vi "Back up values.vi"() -> ()   [LabVIEW 2017]
uses:
  Global/GPIB Type Def.ctl
panel:
  in  "Keithley Values":T1={"range (auto:0)"=0, "range value (volts)"=1000.0, "resolution (4.5 digits:3)"=3, "integration time (0:auto)"=0, "integ. value"=0.01667, "digital filter (off:0)"=0, "advanced filter (off:0)"=0, "dig. filter count"=10.0, "reference (off:0)"=0, "reference value (volts)"=0.0, "noise tolerance (%)"=1.0} {"noise tolerance (%)" min=0.0 max=100.0 step=1.0 format="%^.2e"; "reference value (volts)" min=-1100.0 max=1100.0 format="%^.2e"; "reference (off:0)" items=["off", "set reference value"]; "dig. filter count" min=1.0 max=100.0 step=1.0 format="%^.2e"; "advanced filter (off:0)" items=["off", "enabled"]; "digital filter (off:0)" items=["off", "auto filter", "auto filter once", "moving filter", "repeating filter"]; "integ. value" format="%^.2e"; "integration time (0:auto)" items=["automatic", "automatic once", "set to minimum", "set to maximum", "set aperature value", "set NPLC value"]; "resolution (4.5 digits:3)" items=["auto resolution", "auto resolution once", "3.5 digits", "4.5 digits", "5.5 digits", "6.5 digits", "7.5 digits", "8.5 digits"]; "range (auto:0)" items=["autorange", "autorange once", "set min range", "set max range", "set range value"]; "range value (volts)" min=0.2 max=1000.0 format="%^.2e"}
  in  "Cluster of class private data":T3={"Keithley Multimeter"={"Name"="Keithley Multimeter", "bus"=0.0, "GPIB"=18.0, "GPIB as string"="18", "byte"=1024, "VISA Resource Name"="GPIB0::18::INSTR"}, "Configuration Values"={"range (auto:0)"=0, "dig. filter count"=10.0, "digital filter (off:0)"=0, "advanced filter (off:0)"=0, "integration time (0:auto)"=0, "integ. value"=0.01667, "resolution (4.5 digits:3)"=3, "noise tolerance (%)"=1.0, "reference (off:0)"=0, "coupling"=TRUE, "function (Vdc:1)"=1}, "Frequency Configuration"={"source"=FALSE, "resolution (5 digits:1)"=1, "threshold current range (1mA:0)"=0, "reference value (Hz)"=0.0, "threshold current level"=0.0, "threshold voltage range (10V:1)"=1, "threshold voltage level"=0.0}, "DC Current Configuration"={"reference value (amps)"=0.0, "method"=TRUE, "range value (amps)"=2.0}, "AC Current Configuration"={"detector (rms:0)"=0, "reference value (amps)"=0.0, "range value (amps)"=2.0}, "4 Wire Resistance Configuration"={"offset compensation"=FALSE, "reference value (ohms)"=0.0, "range value (ohms)"=200000.0}, "2 Wire Resistance Configuration"={"offset compensation"=FALSE, "reference value (ohms)"=0.0, "range value (ohms)"=1000000000.0}, "DC Voltage Configuration"={"reference value (volts)"=0.0, "range value (volts)"=1000.0}, "AC Voltage Configuration"={"dBm ref impedance (75:1)"=1, "peak window (secs)"=0.1, "detector (rms:0)"=0, "dB reference (volts)"=1.0, "AC voltage (volts:0)"=0, "reference value (volts)"=0.0, "range value (volts)"=750.0}} {"AC Voltage Configuration"."range value (volts)" min=0.2 max=750.0 format="%^.2e"; "AC Voltage Configuration"."reference value (volts)" min=-775.0 max=775.0 format="%^.2e"; "AC Voltage Configuration"."AC voltage (volts:0)" items=["volts", "DB", "DBM"]; "AC Voltage Configuration"."dB reference (volts)" min=0.001 max=750.0 format="%.3f"; "AC Voltage Configuration"."detector (rms:0)" items=["RMS", "average", "low frequency RMS", "AC peak voltage", "DC negative peak spike", "DC positive peak spike"]; "AC Voltage Configuration"."peak window (secs)" min=0.1 max=9.9 format="%.2f"; "AC Voltage Configuration"."dBm ref impedance (75:1)" items=["50 ohms", "75 ohms", "93 ohms", "132 ohms", "300 ohms", "600 ohms"]; "DC Voltage Configuration"."range value (volts)" min=0.2 max=1000.0 format="%^.2e"; "DC Voltage Configuration"."reference value (volts)" min=-1100.0 max=1100.0 format="%^.2e"; "2 Wire Resistance Configuration"."range value (ohms)" min=20.0 max=1000000000.0 format="%^.2e"; "2 Wire Resistance Configuration"."reference value (ohms)" min=-1000000000.0 max=1000000000.0 format="%^.2e"; "4 Wire Resistance Configuration"."range value (ohms)" min=20.0 max=200000.0 format="%^.2e"; "4 Wire Resistance Configuration"."reference value (ohms)" min=-200000.0 max=200000.0 format="%^.2e"; "AC Current Configuration"."range value (amps)" min=0.0002 max=2.0 format="%^.2e"; "AC Current Configuration"."reference value (amps)" min=-2.1 max=2.1 format="%^.2e"; "AC Current Configuration"."detector (rms:0)" items=["RMS", "average"]; "DC Current Configuration"."range value (amps)" min=0.0002 max=2.0 format="%^.2e"; "DC Current Configuration"."reference value (amps)" min=-2.1 max=2.1 format="%^.2e"; "Frequency Configuration"."threshold voltage level" min=-600.0 max=600.0 step=1.0 format="%^.2e"; "Frequency Configuration"."threshold voltage range (10V:1)" items=["1 V", "10 V", "100 V", "1000 V", "TTL"]; "Frequency Configuration"."threshold current level" min=-0.6 max=0.6 format="%^.2e"; "Frequency Configuration"."reference value (Hz)" min=0.0 max=15000000.0 format="%^.2e"; "Frequency Configuration"."threshold current range (1mA:0)" items=["1 mA", "10 mA", "100 mA", "1 A"]; "Frequency Configuration"."resolution (5 digits:1)" items=["4 digits", "5 digits"]; "Configuration Values"."function (Vdc:1)" items=["ac voltage", "dc voltage", "2-wire resistance", "4-wire resistance", "ac current", "dc current", "frequency", "temperature"]; "Configuration Values"."reference (off:0)" items=["off", "set reference value"]; "Configuration Values"."noise tolerance (%)" min=0.0 max=100.0 step=1.0 format="%^.2e"; "Configuration Values"."resolution (4.5 digits:3)" items=["auto resolution", "auto resolution once", "3.5 digits", "4.5 digits", "5.5 digits", "6.5 digits", "7.5 digits", "8.5 digits"]; "Configuration Values"."integ. value" format="%^.2e"; "Configuration Values"."integration time (0:auto)" items=["automatic", "automatic once", "set to minimum", "set to maximum", "set aperature value", "set NPLC value"]; "Configuration Values"."advanced filter (off:0)" items=["off", "enabled"]; "Configuration Values"."digital filter (off:0)" items=["off", "auto filter", "auto filter once", "moving filter", "repeating filter"]; "Configuration Values"."dig. filter count" min=1.0 max=100.0 step=1.0 format="%^.2e"; "Configuration Values"."range (auto:0)" items=["autorange", "autorange once", "set min range", "set max range", "set range value"]}
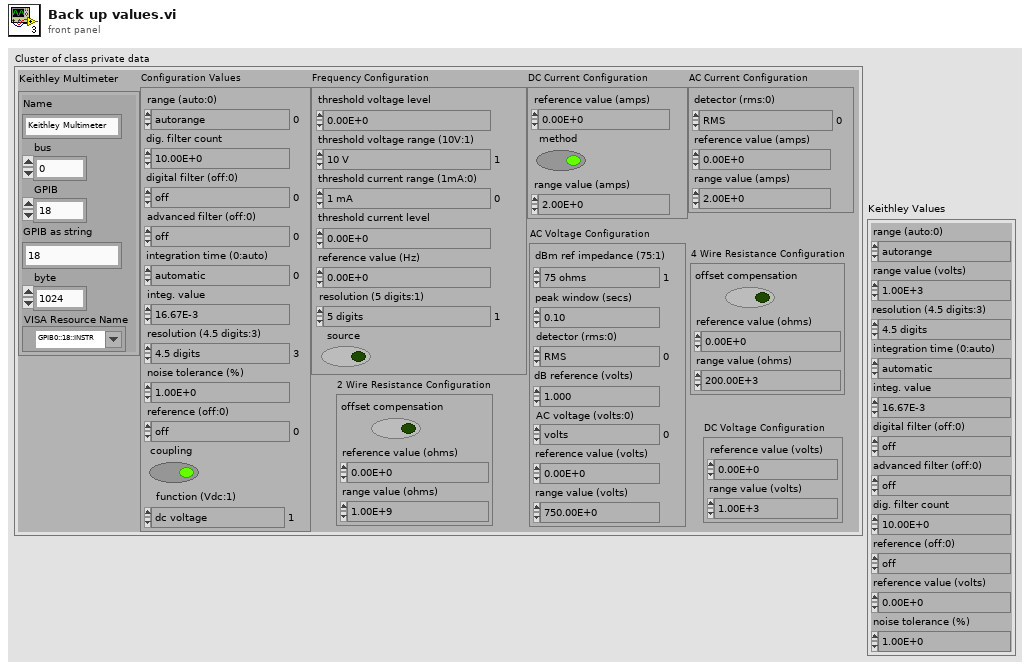
[diagram p1: front panel]
types:
  T1 = cluster{"range (auto:0)":u16, "range value (volts)":dbl, "resolution (4.5 digits:3)":u16, "integration time (0:auto)":u16, "integ. value":dbl, "digital filter (off:0)":u16, "advanced filter (off:0)":u16, "dig. filter count":dbl, "reference (off:0)":u16, "reference value (volts)":dbl, "noise tolerance (%)":dbl}
  T2 = typedef "GPIB Type Def.ctl" = cluster{"Name":string, "bus":dbl, "GPIB":dbl, "GPIB as string":string, "byte":i32, "VISA Resource Name":refnum<visa-resource-name>}
  T3 = cluster{"Keithley Multimeter":T2, "Configuration Values":cluster{"range (auto:0)":u16, "dig. filter count":dbl, "digital filter (off:0)":u16, "advanced filter (off:0)":u16, "integration time (0:auto)":u16, "integ. value":dbl, "resolution (4.5 digits:3)":u16, "noise tolerance (%)":dbl, "reference (off:0)":u16, "coupling":bool, "function (Vdc:1)":u16}, "Frequency Configuration":cluster{"source":bool, "resolution (5 digits:1)":u16, "threshold current range (1mA:0)":u16, "reference value (Hz)":dbl, "threshold current level":dbl, "threshold voltage range (10V:1)":u16, "threshold voltage level":dbl}, "DC Current Configuration":cluster{"reference value (amps)":dbl, "method":bool, "range value (amps)":dbl}, "AC Current Configuration":cluster{"detector (rms:0)":u16, "reference value (amps)":dbl, "range value (amps)":dbl}, "4 Wire Resistance Configuration":cluster{"offset compensation":bool, "reference value (ohms)":dbl, "range value (ohms)":dbl}, "2 Wire Resistance Configuration":cluster{"offset compensation":bool, "reference value (ohms)":dbl, "range value (ohms)":dbl}, "DC Voltage Configuration":cluster{"reference value (volts)":dbl, "range value (volts)":dbl}, "AC Voltage Configuration":cluster{"dBm ref impedance (75:1)":u16, "peak window (secs)":dbl, "detector (rms:0)":u16, "dB reference (volts)":dbl, "AC voltage (volts:0)":u16, "reference value (volts)":dbl, "range value (volts)":dbl}}
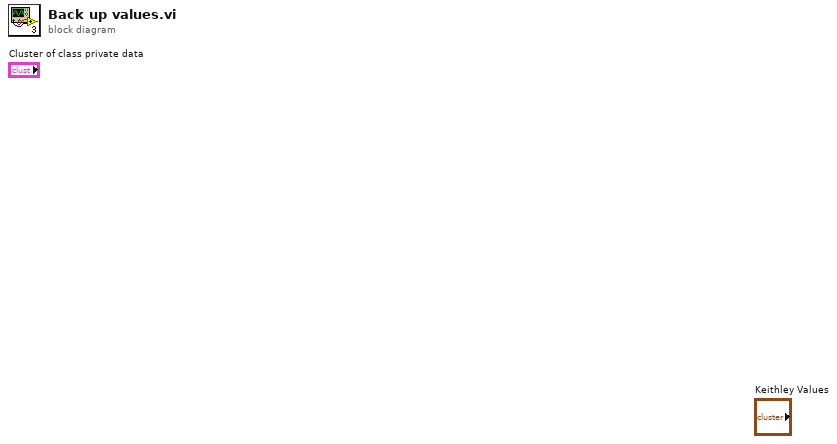
[diagram p0: block diagram]
diagram:
